vi "16TILMMonitor.vi"() -> ()   [LabVIEW 2019]
uses:
  Global/Global Variables/Data_Display_global.vi
  Instrument_Setup.vi
  Utility/Monitor Communication/sub-vis/ILM_Check_Queue.vi
  Utility/Monitor Communication/sub-vis/ILM_Open_Queue.vi
  Equipment/Mercury iXX/Mercury iXX.lvlib
  Equipment/Mercury iXX/Public/Libraries/Level Meter.lvlib
  Equipment/Mercury iXX/Public/Libraries/Level Meter/Open/Open Level Meter Device.vi
  Equipment/Mercury iXX/Public/Libraries/Level Meter/Signals/Read/Probe Level Helium (Read).vi
  Utility/Monitor Communication/S16/ILM-Cluster.ctl
panel:
  out "ILM":T1 {"Nitrogen" format="%#4_5f"}
  # "N (%)"
  # "He (%)"
  # "Levelmeter"
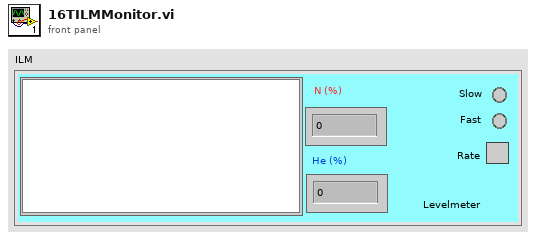
[diagram p1: front panel]
types:
  T1 = typedef "ILM-Cluster.ctl" = cluster{"Plot":dbl[][], "Nitrogen":dbl, "Helium":dbl, "Fast":bool, "Slow":bool, "Rate":bool}
  T2 = typedef "Mercury iXX.lvlib/Mercury Reference.ctl" = cluster{"Comms":refnum<visa-resource-name>, "Device ID":string[], "Comms Layer":T3, "Command":string, "Query reference":T4}
  T3 = typedef "Mercury iXX.lvlib/Comms Transport Layer.ctl" = enum16{"Ethernet TCP/IP", "USB", "ISOBus - RS-232", "GPIB"}
  T4 = typedef "Mercury iXX.lvlib/Query Dynamic Reference.ctl" = refnum<vi>
  T5 = typedef "ILM-Control.ctl" = cluster{"Rate":bool}
  T6 = cluster{"Sensor Length (cm)":sgl, "Hi Setpoint (cm)":sgl, "Lo Setpoint (cm)":sgl, "Sampling Interval (min)":sgl}
  T7 = cluster{"error":bool, "code":i32, "source":string}
  T8 = cluster{"Display Channel":i32[], "Instrument address":cluster{"Com Port":i32, "ISOBUS Address":i32, "GPIB Address":i16, "Communication":enum16{"RS232", "ISOBUS", "GPIB", "Gateway"}}}
  T9 = cluster{"Com Port":i32, "ISOBUS Address":i32, "GPIB Address":i16, "Communication":enum16{"RS232", "ISOBUS", "GPIB", "Gateway"}}
  T10 = typedef "ILMChannelStatus.ctl" = cluster{"Probe current":bool, "Probe fast":bool, "Probe slow":bool, "Auto-fill":enum16{"End fill", "Not filling", "Filling", "Start filling"}, "Fill":bool, "Low level":bool, "Alm requested":bool, "Pre-pulse I":bool}
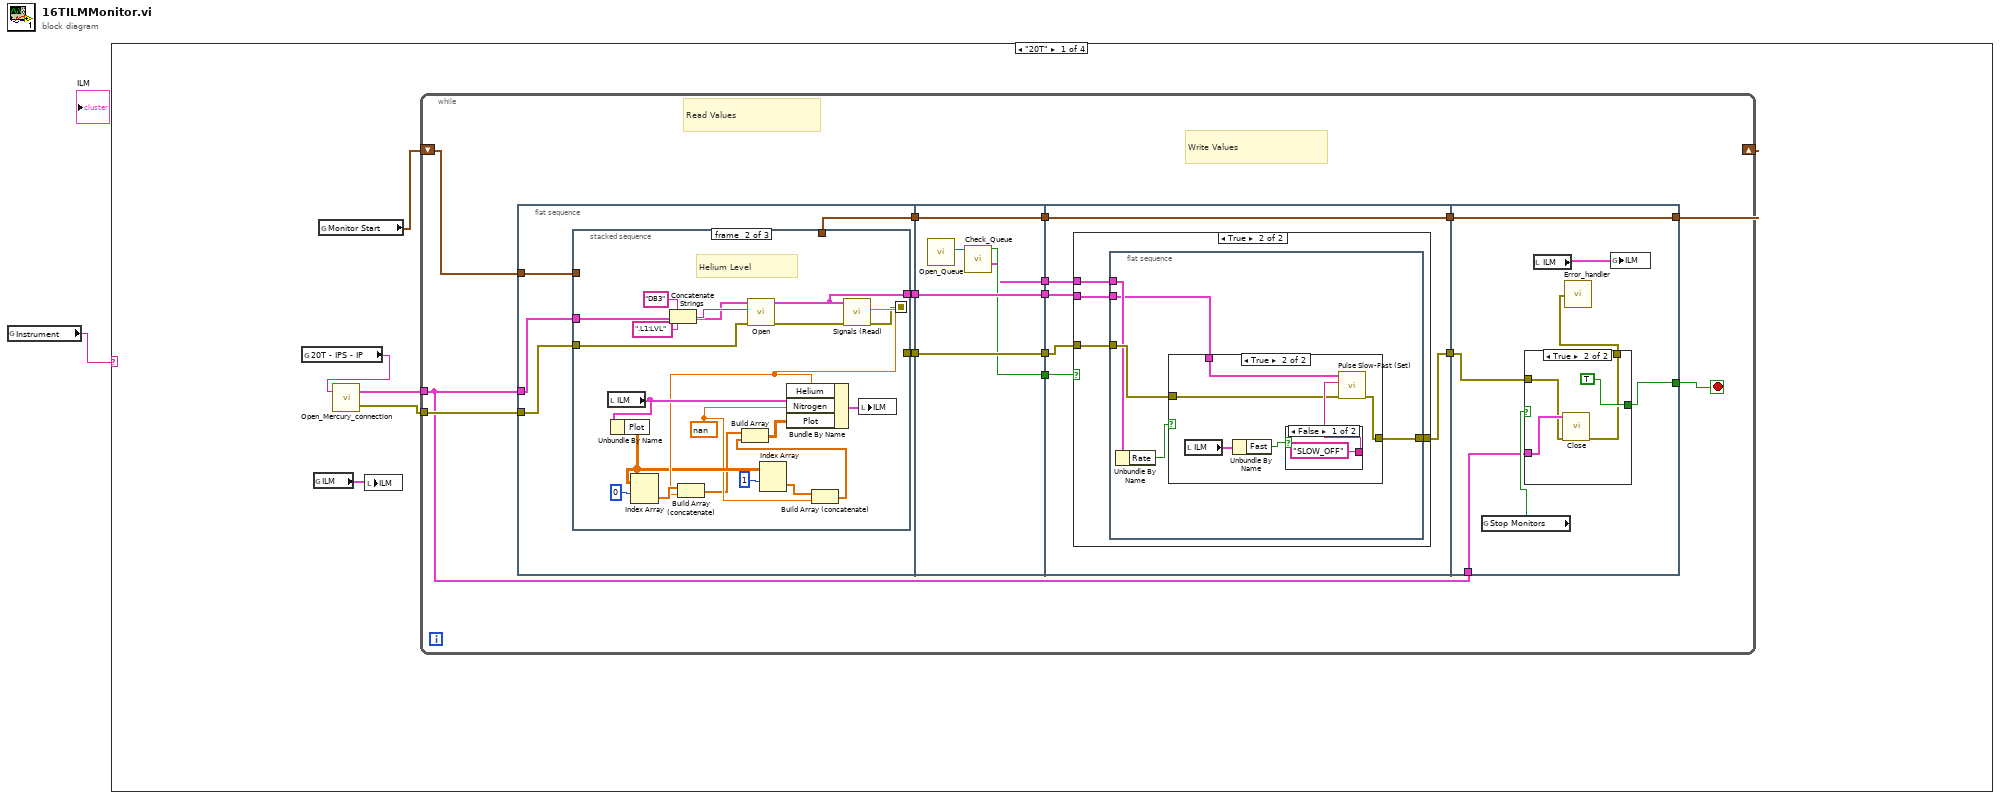
[diagram p0: block diagram]
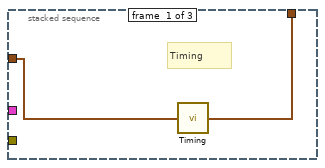
[diagram p2: hidden frame]
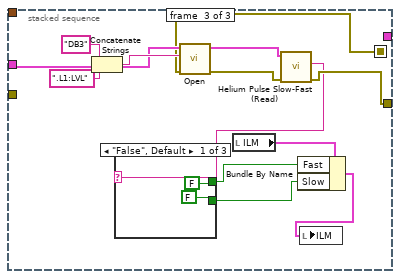
[diagram p3: hidden frame]
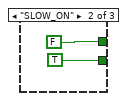
[diagram p4: hidden frame]
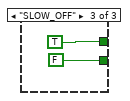
[diagram p5: hidden frame]
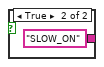
[diagram p8: hidden frame]
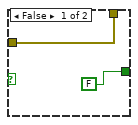
[diagram p9: hidden frame]
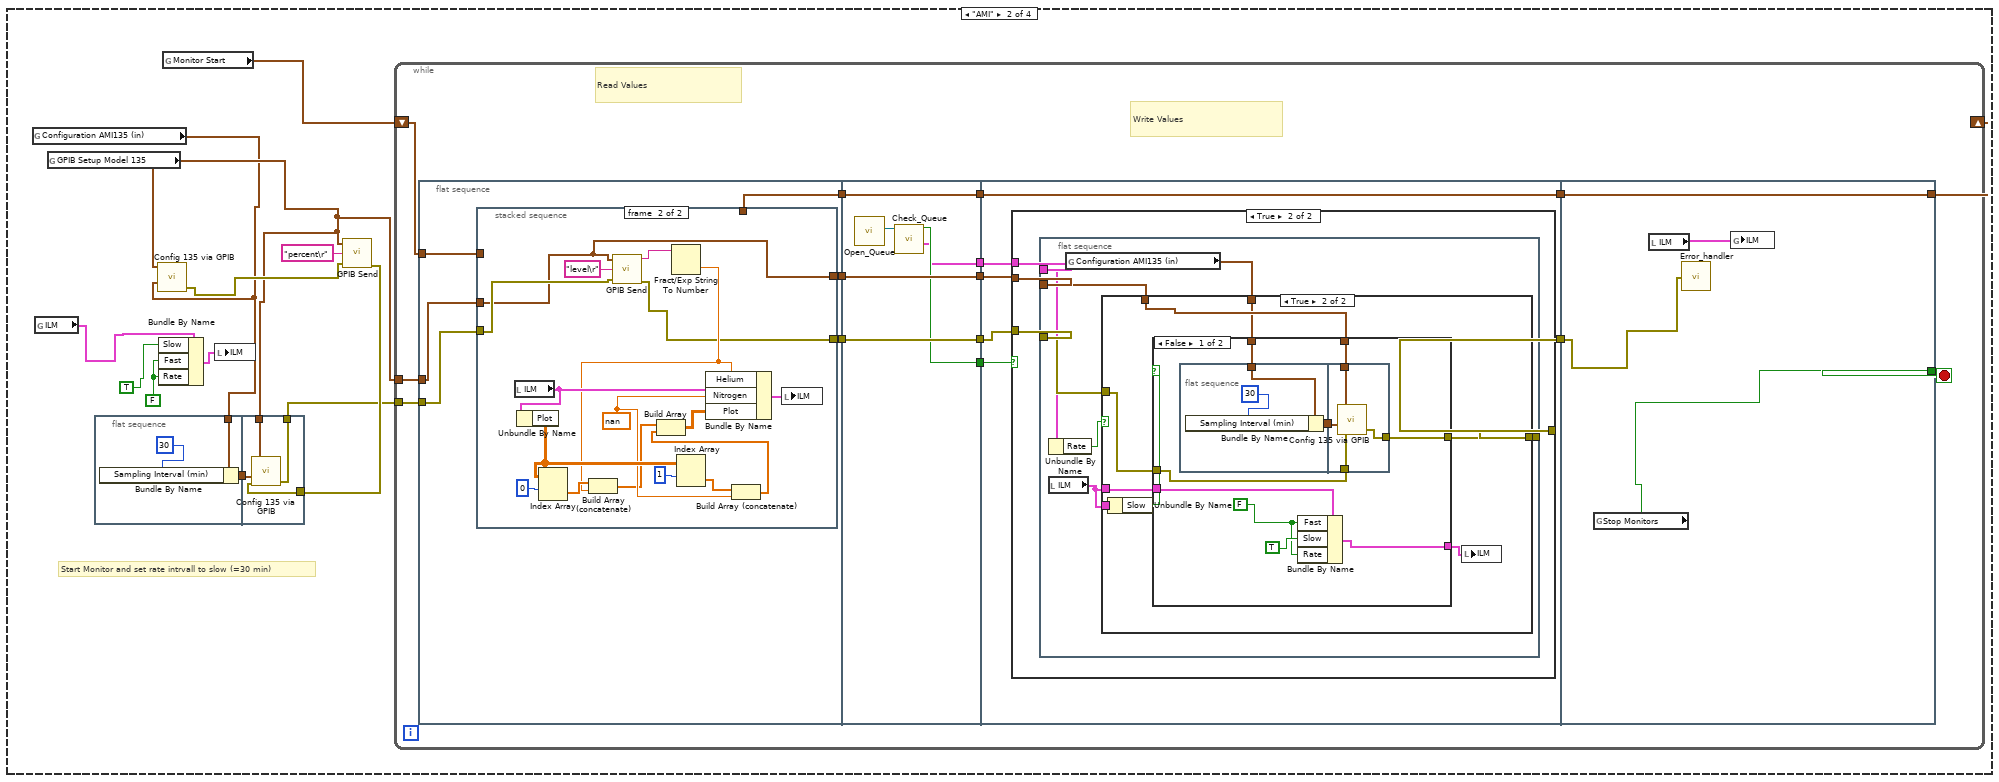
[diagram p10: hidden frame]
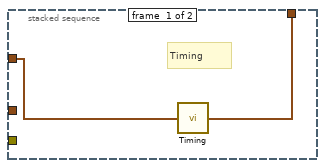
[diagram p11: hidden frame]
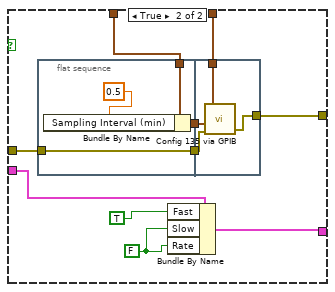
[diagram p14: hidden frame]
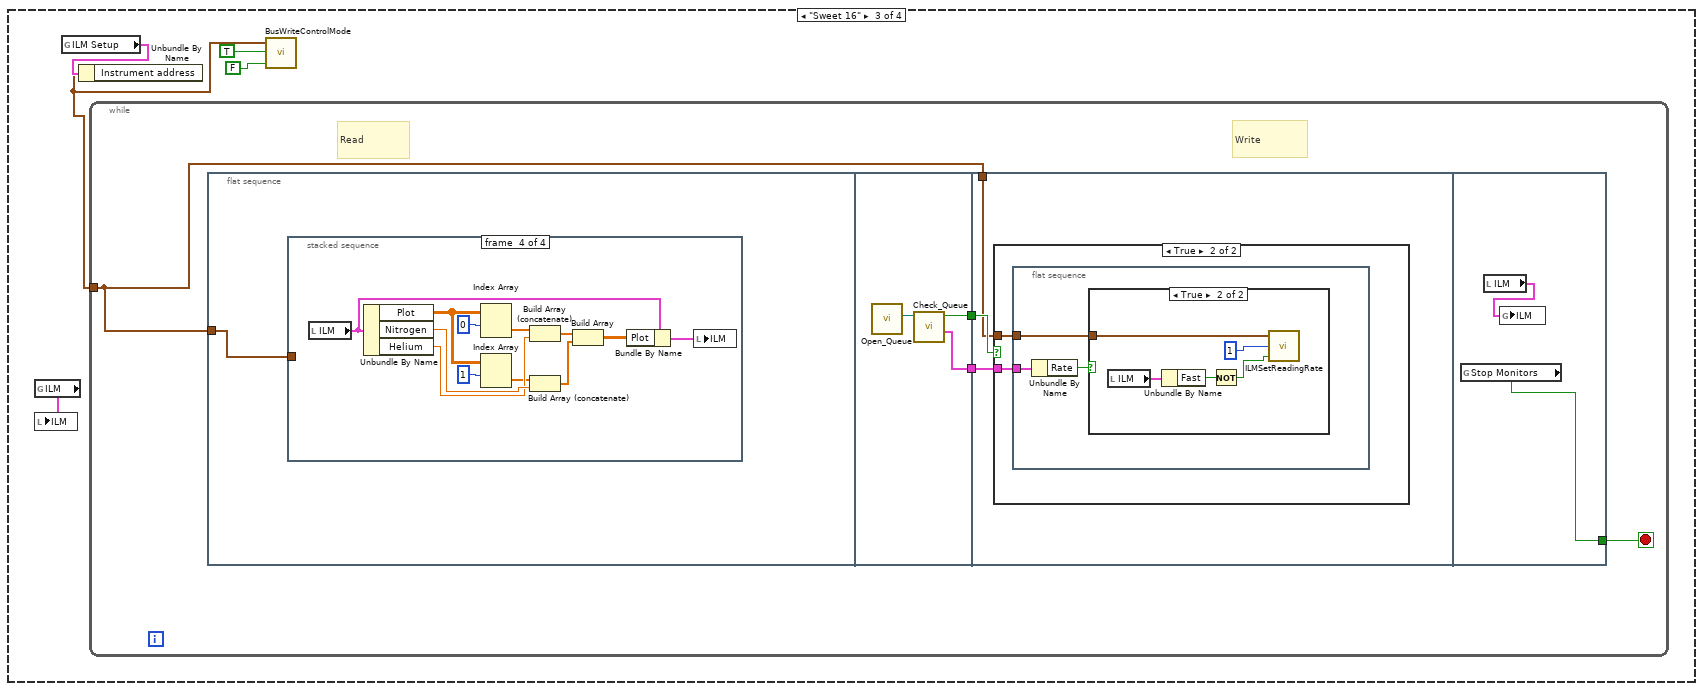
[diagram p15: hidden frame]
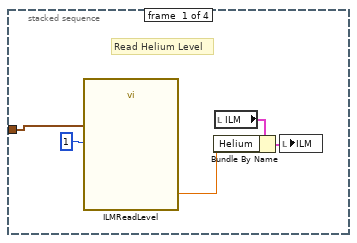
[diagram p16: hidden frame]
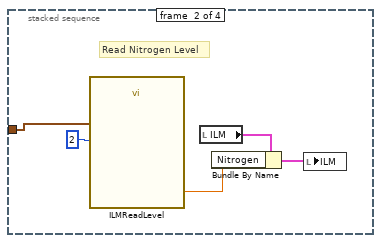
[diagram p17: hidden frame]
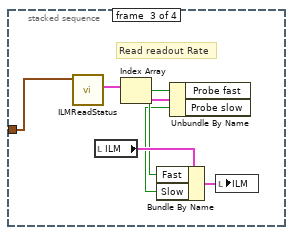
[diagram p18: hidden frame]
diagram:
  n1 = global read "Instrument_Setup.vi" "Instrument"() -> (w1:string)
  n2 = case shown="\"20T\"" w1 {
    frame "20T" {
      n3 = global read "Instrument_Setup.vi" "20T - IPS - IP"() -> (w4:string)
      n4 = global read "Data_Display_global.vi" "ILM"() -> (w2:T1)
      n5 = global read "Data_Display_global.vi" "Monitor Start"() -> (w3:timestamp)
      n6 = call "Open_Mercury_connection.vi"("IP Address"=w4) -> ("error out"=w5:errorcluster, "Mercury Reference Out"=w6:T2)  [unwired: 1 in]
      n7 = local write "ILM"(w2) -> ()
      n8 = while {
        tunnel: w6 -> [w10]
        tunnel: w5 -> [w21]
        shift-right: [w19] -> _
        shift-left: w3 -> [w20]
        stop <- w7 stop-if-true
        # "Read Values"
        # "Write Values"
        n9 = flat-sequence {
          tunnel: w21 -> [w27]
          tunnel: w10 -> [w26]
          tunnel: w20 -> [w25]
          tunnel: [w24] -> w18
          tunnel: [w22] -> w17
          tunnel: [w23] -> w16
          tunnel: w18 -> [w74]
          tunnel: w17 -> [w73]
          tunnel: w16 -> [w72]
          tunnel: [w74] -> w15
          tunnel: [w73] -> w14
          tunnel: [w72] -> w13
          tunnel: [w70] -> w9
          tunnel: [w69] -> w8
          tunnel: w15 -> [w80]
          tunnel: w14 -> [w76]
          tunnel: w13 -> [w77]
          tunnel: [w80] -> w12
          tunnel: [w75] -> w11
          tunnel: w9 -> [w79]
          tunnel: w8 -> [w78]
          tunnel: [w106] -> w19
          tunnel: w12 -> [w106]
          tunnel: w11 -> [w102]
          tunnel: w10 -> [w103]
          tunnel: [w100] -> w7
          frame #0 {
            n10 = stacked-sequence {
              seq-local: [_ w30 _] -> [_ _ w58]
              tunnel: w26 -> [_ w45 w59]
              tunnel: w27 -> [_ w44 _]
              tunnel: w25 -> [w29 _ _]
              tunnel: [w28 _ _] -> w24
              tunnel: [_ w42 _] -> w23
              tunnel: [_ _ w55] -> w22
              frame #0 {
                # "Timing"
                n11 = call "Timing.vi"("start time (s)"=w29) -> ("last reading (s)"=w28:timestamp)
              }
              frame #1 {
                w34 = nan
                # "Helium Level"
                n12 = local read "ILM"() -> (w39:T1)
                n13 = Unbundle By Name(w39) -> ("Plot"=w36:dbl[][])
                n14 = Index Array(array=w36, index (row)=0 ("index")) -> (element=w40:dbl[])  [unwired: 1 in]
                n15 = Concatenate Strings("DB3", ".L1:LVL" ("Device Identifier")) -> (w48:string)
                n16 = call-poly "Open.vi"("error in (no error)"=w44, "Device Identifier"=w48, "Mercury Reference In"=w45) -> ("error out"=w49:errorcluster, "Mercury Reference Out"=w42:T2)  [unwired: 1 in, 6 out]
                n17 = Index Array(array=w36, index (row)=1 ("index")) -> (element=w35:dbl[])  [unwired: 1 in]
                n18 = Build Array (concatenate)(w35, w34) -> (w32:dbl[])
                n19 = call-poly "Signals (Read).vi"("error in"=w49, "Mercury Reference In"=w42) -> ("error out"=w30:errorcluster, "Level"=w38:dbl)  [unwired: 5 in, 3 out]
                n20 = Build Array (concatenate)(w40, w38) -> (w33:dbl[])
                n21 = Build Array(w33, w32) -> (w31:dbl[][])
                n22 = Bundle By Name(cluster=w39, "Helium"=w38, "Nitrogen"=w34, "Plot"=w31) -> (w43:T1)
                n23 = local write "ILM"(w43) -> ()
              }
              frame #2 {
                n24 = Concatenate Strings("DB3", ".L1:LVL" ("Device Identifier")) -> (w62:string)
                n25 = call-poly "Open.vi"("error in (no error)"=w58, "Device Identifier"=w62, "Mercury Reference In"=w59) -> ("error out"=w56:errorcluster, "Mercury Reference Out"=w57:T2)  [unwired: 1 in, 6 out]
                n26 = local read "ILM"() -> (w53:T1)
                n27 = call "Helium Pulse Slow-Fast (Read).vi"("error in"=w56, "Mercury Reference In"=w57) -> ("error out"=w55:errorcluster, "Response"=w54:string)  [unwired: 6 in, 2 out]
                n28 = case shown="\"False\", Default" w54 {
                  tunnel: [FALSE FALSE TRUE] -> w52
                  tunnel: [FALSE TRUE FALSE] -> w51
                  frame "False", Default {
                  }
                  frame "SLOW_ON" {
                  }
                  frame "SLOW_OFF" {
                  }
                }
                n29 = Bundle By Name(cluster=w53, "Fast"=w52, "Slow"=w51) -> (w50:T1)
                n30 = local write "ILM"(w50) -> ()
              }
            }
          }
          frame #1 {
            n31 = call-poly "Open_Queue.vi"() -> ("queue out"=w71:refnum<queue>)  [unwired: 10 in, 1 out]
            n32 = call-poly "Check_Queue.vi"("queue"=w71) -> ("SR830-2 2"=w69:T5, "New Entries?"=w70:bool)  [unwired: 7 in, 1 out]
          }
          frame #2 {
            n33 = case shown="True" w79 {
              tunnel: w76 -> [w81 w82]
              tunnel: w77 -> [_ w85]
              tunnel: w78 -> [_ w84]
              tunnel: [w81 w83] -> w75
              frame False {
              }
              frame True {
                n34 = flat-sequence {
                  tunnel: w82 -> [w89]
                  tunnel: w85 -> [w86]
                  tunnel: w84 -> [w87]
                  tunnel: [w88] -> w83
                  frame #0 {
                    n35 = Unbundle By Name(w87) -> ("Rate"=w90:bool)
                    n36 = case shown="True" w90 {
                      tunnel: w86 -> [_ w96]
                      tunnel: w89 -> [w91 w93]
                      tunnel: [w91 w92] -> w88
                      frame False {
                      }
                      frame True {
                        n37 = local read "ILM"() -> (w97:T1)
                        n38 = Unbundle By Name(w97) -> ("Fast"=w95:bool)
                        n39 = case shown="False" w95 {
                          tunnel: ["SLOW_OFF" "SLOW_ON"] -> w94
                          frame False {
                          }
                          frame True {
                          }
                        }
                        n40 = call "Pulse Slow-Fast (Set).vi"("error in"=w93, "Delay"=w94, "Mercury Reference In"=w96) -> ("error out"=w92:errorcluster)  [unwired: 5 in, 3 out]
                      }
                    }
                  }
                }
              }
            }
          }
          frame #3 {
            n41 = global read "Data_Display_global.vi" "Stop Monitors"() -> (w104:bool)
            n42 = case shown="True" w104 {
              tunnel: w103 -> [_ w112]
              tunnel: [FALSE TRUE] -> w100
              tunnel: w102 -> [w107 w109]
              tunnel: [w107 w110] -> w101
              frame False {
              }
              frame True {
                n43 = call "Close.vi"("error in (no error)"=w109, "Mercury Reference"=w112) -> ("error out"=w110:errorcluster)  [unwired: 9 in]
              }
            }
            n44 = local read "ILM"() -> (w105:T1)
            n45 = call "Error_handler.vi"("error constant"=w101) -> ()
            n46 = global write "Data_Display_global.vi" "ILM"(w105) -> ()
          }
        }
      }
    }
    frame "AMI" {
      w113 = FALSE
      # "Start Monitor and set rate intrvall to slow (=30 min)"
      n47 = global read "Instrument_Setup.vi" "Configuration AMI135 (in)"() -> (w119:T6)
      n48 = global read "Data_Display_global.vi" "ILM"() -> (w115:T1)
      n49 = global read "Instrument_Setup.vi" "GPIB Setup Model 135"() -> (w120:cluster{"GPIB address":i16, "GPIB bus":i16})
      n50 = flat-sequence {
        tunnel: w119 -> [w126]
        tunnel: [w125] -> w121
        tunnel: w121 -> [w131]
        tunnel: w120 -> [w130]
        tunnel: w118 -> [w129]
        tunnel: [w128] -> w117
        frame #0 {
          n51 = Bundle By Name(cluster=w126, "Sampling Interval (min)"=30) -> (w125:T6)
        }
        frame #1 {
          n52 = call "Config 135 via GPIB.vi"("error in"=w129, "Configuration (in)"=w131, "GPIB Setup"=w130) -> ("error out"=w128:T7)  [unwired: 1 in, 2 out]
        }
      }
      n53 = call "Config 135 via GPIB.vi"("Configuration (in)"=w119, "GPIB Setup"=w120) -> ("error out"=w122:T7)  [unwired: 2 in, 2 out]
      n54 = Bundle By Name(cluster=w115, "Slow"=TRUE, "Fast"=w113, "Rate"=w113) -> (w114:T1)
      n55 = global read "Data_Display_global.vi" "Monitor Start"() -> (w124:timestamp)
      n56 = local write "ILM"(w114) -> ()
      n57 = call "GPIB Send.vi"("GPIB Setup"=w120, "Input command"="percent\r", "error in"=w122) -> ("error out"=w118:T7)  [unwired: 3 out]
      n58 = while {
        tunnel: w120 -> [w132]
        tunnel: w117 -> [w146]
        shift-right: [w144] -> _
        shift-left: w124 -> [w145]
        stop <- w133 stop-if-true
        # "Read Values"
        # "Write Values"
        n59 = flat-sequence {
          tunnel: w146 -> [w152]
          tunnel: w132 -> [w151]
          tunnel: w145 -> [w150]
          tunnel: [w149] -> w143
          tunnel: [w147] -> w142
          tunnel: [w148] -> w141
          tunnel: w143 -> [w177]
          tunnel: w142 -> [w176]
          tunnel: w141 -> [w175]
          tunnel: [w177] -> w140
          tunnel: [w176] -> w139
          tunnel: [w175] -> w138
          tunnel: [w173] -> w135
          tunnel: [w172] -> w134
          tunnel: w140 -> [w183]
          tunnel: w139 -> [w179]
          tunnel: w138 -> [w180]
          tunnel: [w183] -> w137
          tunnel: [w178] -> w136
          tunnel: w135 -> [w182]
          tunnel: w134 -> [w181]
          tunnel: [w242] -> w144
          tunnel: w137 -> [w242]
          tunnel: w136 -> [w239]
          tunnel: [w240] -> w133
          frame #0 {
            n60 = stacked-sequence {
              tunnel: w151 -> [_ w156]
              tunnel: w152 -> [_ w158]
              tunnel: w150 -> [w154 _]
              tunnel: [w153 _] -> w149
              tunnel: [_ w156] -> w148
              tunnel: [_ w155] -> w147
              frame #0 {
                # "Timing"
                n61 = call "Timing.vi"("start time (s)"=w154) -> ("last reading (s)"=w153:timestamp)
              }
              frame #1 {
                w164 = nan
                n62 = local read "ILM"() -> (w168:T1)
                n63 = Unbundle By Name(w168) -> ("Plot"=w166:dbl[][])
                n64 = Index Array(array=w166, index (row)=0 ("index")) -> (element=w169:dbl[])  [unwired: 1 in]
                n65 = call "GPIB Send.vi"("GPIB Setup"=w156, "Input command"="level\r", "error in"=w158) -> ("Return string"=w159:string, "error out"=w155:T7)  [unwired: 2 out]
                n66 = Fract/Exp String To Number(string=w159) -> (number=w157:dbl)  [unwired: 3 in, 1 out]
                n67 = Build Array (concatenate)(w169, w157) -> (w163:dbl[])
                n68 = Index Array(array=w166, index (row)=1 ("index")) -> (element=w165:dbl[])  [unwired: 1 in]
                n69 = Build Array (concatenate)(w165, w164) -> (w162:dbl[])
                n70 = Build Array(w163, w162) -> (w161:dbl[][])
                n71 = Bundle By Name(cluster=w168, "Helium"=w157, "Nitrogen"=w164, "Plot"=w161) -> (w171:T1)
                n72 = local write "ILM"(w171) -> ()
              }
            }
          }
          frame #1 {
            n73 = call-poly "Open_Queue.vi"() -> ("queue out"=w174:refnum<queue>)  [unwired: 10 in, 1 out]
            n74 = call-poly "Check_Queue.vi"("queue"=w174) -> ("SR830-2 2"=w172:T5, "New Entries?"=w173:bool)  [unwired: 7 in, 1 out]
          }
          frame #2 {
            n75 = case shown="True" w182 {
              tunnel: w179 -> [w184 w185]
              tunnel: w180 -> [_ w188]
              tunnel: w181 -> [_ w187]
              tunnel: [w184 w186] -> w178
              frame False {
              }
              frame True {
                n76 = flat-sequence {
                  tunnel: w185 -> [w194]
                  tunnel: w188 -> [w191]
                  tunnel: w187 -> [w192]
                  tunnel: [w193] -> w186
                  frame #0 {
                    n77 = Unbundle By Name(w192) -> ("Rate"=w195:bool)
                    n78 = local read "ILM"() -> (w189:T1)
                    n79 = global read "Instrument_Setup.vi" "Configuration AMI135 (in)"() -> (w190:T6)
                    n80 = case shown="True" w195 {
                      tunnel: w191 -> [_ w202]
                      tunnel: w194 -> [w196 w197]
                      tunnel: [w196 w198] -> w193
                      tunnel: w189 -> [_ w204]
                      tunnel: w190 -> [_ w201]
                      tunnel: w189 -> [_ w200]
                      frame False {
                      }
                      frame True {
                        n81 = Unbundle By Name(w204) -> ("Slow"=w203:bool)
                        n82 = case shown="False" w203 {
                          tunnel: w202 -> [w212 w229]
                          tunnel: w201 -> [w211 w228]
                          tunnel: w200 -> [w210 w224]
                          tunnel: [w208 w225] -> w199
                          tunnel: [w205 w223] -> w198
                          tunnel: w197 -> [w206 w221]
                          frame False {
                            w207 = FALSE
                            n83 = flat-sequence {
                              tunnel: [w215] -> w213
                              tunnel: w211 -> [w214]
                              tunnel: w213 -> [w220]
                              tunnel: w212 -> [w219]
                              tunnel: w206 -> [w218]
                              tunnel: [w217] -> w205
                              frame #0 {
                                n84 = Bundle By Name(cluster=w214, "Sampling Interval (min)"=30) -> (w215:T6)
                              }
                              frame #1 {
                                n85 = call "Config 135 via GPIB.vi"("error in"=w218, "Configuration (in)"=w220, "GPIB Setup"=w219) -> ("error out"=w217:T7)  [unwired: 1 in, 2 out]
                              }
                            }
                            n86 = Bundle By Name(cluster=w210, "Fast"=w207, "Slow"=TRUE, "Rate"=w207) -> (w208:T1)
                          }
                          frame True {
                            w226 = FALSE
                            n87 = flat-sequence {
                              tunnel: [w233] -> w230
                              tunnel: w228 -> [w232]
                              tunnel: [w231] -> w222
                              tunnel: w221 -> [w231]
                              tunnel: w230 -> [w238]
                              tunnel: w229 -> [w237]
                              tunnel: [w236] -> w223
                              tunnel: w222 -> [w235]
                              frame #0 {
                                n88 = Bundle By Name(cluster=w232, "Sampling Interval (min)"=0.5) -> (w233:T6)
                              }
                              frame #1 {
                                n89 = call "Config 135 via GPIB.vi"("error in"=w235, "Configuration (in)"=w238, "GPIB Setup"=w237) -> ("error out"=w236:T7)  [unwired: 1 in, 2 out]
                              }
                            }
                            n90 = Bundle By Name(cluster=w224, "Fast"=TRUE, "Slow"=w226, "Rate"=w226) -> (w225:T1)
                          }
                        }
                        n91 = local write "ILM"(w199) -> ()
                      }
                    }
                  }
                }
              }
            }
          }
          frame #3 {
            n92 = global read "Data_Display_global.vi" "Stop Monitors"() -> (w240:bool)
            n93 = local read "ILM"() -> (w241:T1)
            n94 = call "Error_handler.vi"("error constant"=w239) -> ()
            n95 = global write "Data_Display_global.vi" "ILM"(w241) -> ()
          }
        }
      }
    }
    frame "Sweet 16" {
      n96 = global read "Data_Display_global.vi" "ILM"() -> (w243:T1)
      n97 = local write "ILM"(w243) -> ()
      n98 = global read "Instrument_Setup.vi" "ILM Setup"() -> (w247:T8)
      n99 = Unbundle By Name(w247) -> ("Instrument address"=w244:T9)
      n100 = while {
        tunnel: w244 -> [w249]
        stop <- w248 stop-if-true
        # "Read"
        # "Write"
        n101 = flat-sequence {
          tunnel: w249 -> [w252]
          tunnel: [w283] -> w251
          tunnel: [w282] -> w250
          tunnel: w251 -> [w287]
          tunnel: w250 -> [w286]
          tunnel: w249 -> [w285]
          tunnel: [w299] -> w248
          frame #0 {
            n102 = stacked-sequence {
              tunnel: w252 -> [w256 w261 w263 _]
              frame #0 {
                # "Read Helium Level"
                n103 = call "ILMReadLevel.vi"("Address"=w256, "Channel number (1-3)"=u8 1) -> ("Level"=w253:dbl)  [unwired: 2 out]
                n104 = local read "ILM"() -> (w255:T1)
                n105 = Bundle By Name(cluster=w255, "Helium"=w253) -> (w254:T1)
                n106 = local write "ILM"(w254) -> ()
              }
              frame #1 {
                # "Read Nitrogen Level"
                n107 = call "ILMReadLevel.vi"("Address"=w261, "Channel number (1-3)"=u8 2) -> ("Level"=w258:dbl)  [unwired: 2 out]
                n108 = local read "ILM"() -> (w260:T1)
                n109 = Bundle By Name(cluster=w260, "Nitrogen"=w258) -> (w259:T1)
                n110 = local write "ILM"(w259) -> ()
              }
              frame #2 {
                # "Read readout Rate"
                n111 = call "ILMReadStatus.vi"("Instrument address"=w263) -> ("Channel"=w268:T10[])  [unwired: 3 in, 3 out]
                n112 = local read "ILM"() -> (w267:T1)
                n113 = Index Array(array=w268) -> (element=w269:T10)  [unwired: 1 in]
                n114 = Unbundle By Name(w269) -> ("Probe fast"=w265:bool, "Probe slow"=w264:bool)
                n115 = Bundle By Name(cluster=w267, "Fast"=w265, "Slow"=w264) -> (w266:T1)
                n116 = local write "ILM"(w266) -> ()
              }
              frame #3 {
                n117 = local read "ILM"() -> (w272:T1)
                n118 = Unbundle By Name(w272) -> ("Plot"=w275:dbl[][], "Nitrogen"=w279:dbl, "Helium"=w278:dbl)
                n119 = Index Array(array=w275, index (row)=0 ("index")) -> (element=w276:dbl[])  [unwired: 1 in]
                n120 = Index Array(array=w275, index (row)=1 ("index")) -> (element=w274:dbl[])  [unwired: 1 in]
                n121 = Build Array (concatenate)(w276, w278) -> (w280:dbl[])
                n122 = Build Array (concatenate)(w274, w279) -> (w281:dbl[])
                n123 = Build Array(w280, w281) -> (w270:dbl[][])
                n124 = Bundle By Name(cluster=w272, "Plot"=w270) -> (w271:T1)
                n125 = local write "ILM"(w271) -> ()
              }
            }
          }
          frame #1 {
            n126 = call-poly "Open_Queue.vi"() -> ("queue out"=w284:refnum<queue>)  [unwired: 10 in, 1 out]
            n127 = call-poly "Check_Queue.vi"("queue"=w284) -> ("SR830-2 2"=w283:T5, "New Entries?"=w282:bool)  [unwired: 7 in, 1 out]
          }
          frame #2 {
            n128 = case shown="True" w286 {
              tunnel: w287 -> [_ w289]
              tunnel: w285 -> [_ w288]
              frame False {
              }
              frame True {
                n129 = flat-sequence {
                  tunnel: w289 -> [w291]
                  tunnel: w288 -> [w292]
                  frame #0 {
                    n130 = Unbundle By Name(w291) -> ("Rate"=w290:bool)
                    n131 = case shown="True" w290 {
                      tunnel: w292 -> [_ w296]
                      frame False {
                      }
                      frame True {
                        n132 = local read "ILM"() -> (w295:T1)
                        n133 = Unbundle By Name(w295) -> ("Fast"=w294:bool)
                        n134 = Not(x=w294) -> (.not. x?=w293:bool)
                        n135 = call "ILMSetReadingRate.vi"("Fast"=w293, "Channel(1-3)"=1, "Address"=w296) -> ()  [unwired: 1 out]
                      }
                    }
                  }
                }
              }
            }
          }
          frame #3 {
            n136 = global read "Data_Display_global.vi" "Stop Monitors"() -> (w299:bool)
            n137 = local read "ILM"() -> (w298:T1)
            n138 = global write "Data_Display_global.vi" "ILM"(w298) -> ()
          }
        }
      }
      n139 = call "BusWriteControlMode.vi"("Locked"=FALSE, "Remote"=TRUE, "Address"=w244) -> ()  [unwired: 1 out]
    }
    frame "empty", Default {
    }
  }
